vi "Solution part 1.vi"(11 "data?":bool) -> (3 "Distance":i32)   [LabVIEW 2020]
uses:
  Direction.ctl
  WindStar.ctl
panel:
  out "Non-90deg turn!":bool
  out "Last parsed line":i32
  out "Direction":T1
  out "Position":T2
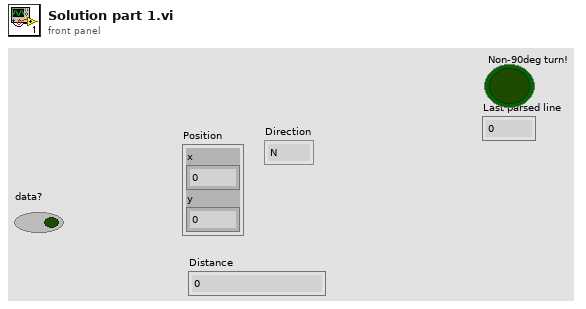
[diagram p1: front panel]
types:
  T1 = typedef "WindStar.ctl" = enum16{"N", "NE", "E", "SE", "S", "SW", "W", "NW", "F", "R", "L"}
  T2 = typedef "Direction.ctl" = cluster{"x":i32, "y":i32}
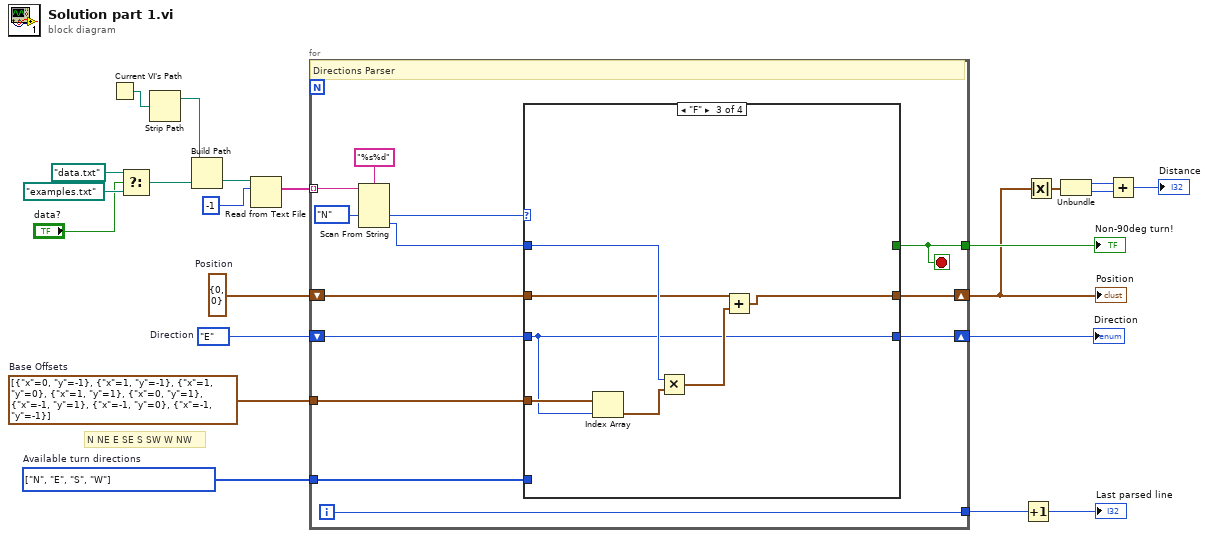
[diagram p0: block diagram]
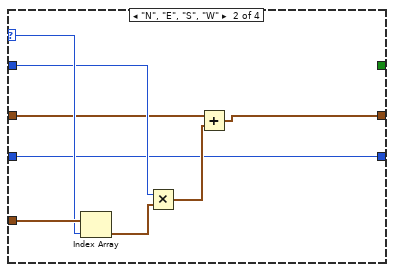
[diagram p3: hidden frame]
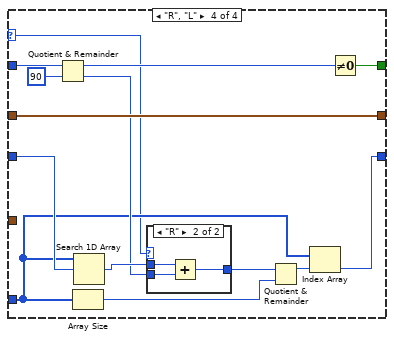
[diagram p4: hidden frame]
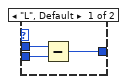
[diagram p5: hidden frame]
diagram:
  w9 = T1[] [enum."N", enum."E", enum."S", enum."W"] items=["N", "NE", "E", "SE", "S", "SW", "W", "NW", "F", "R", "L"]  # Available turn directions
  w13 = WindStar."E"  # Direction
  w11 = T2[] [{"x"=0, "y"=-1}, {"x"=1, "y"=-1}, {"x"=1, "y"=0}, {"x"=1, "y"=1}, {"x"=0, "y"=1}, {"x"=-1, "y"=1}, {"x"=-1, "y"=0}, {"x"=-1, "y"=-1}]  # Base Offsets
  w12 = T2 {"x"=0, "y"=0}  # Position
  # "N NE E SE S SW W NW"
  n1 = Current VI's Path() -> (path=w19:path)
  n2 = Select(t=path "data.txt", s="data?", f=path "examples.txt") -> (s? t:f=w20:path)
  n3 = Strip Path(path=w19) -> (stripped path=w18:path)  [unwired: 1 out]
  n4 = Build Path(base path=w18, name or relative path=w20) -> (appended path=w17:path)
  n5 = Read from Text File(file (use dialog)=w17, count=-1) -> (text=w14:string[])  [unwired: 2 in, 3 out]
  n6 = for {
    tunnel: w14 -> [w35] mode=indexing
    shift-right: [w28] -> w10
    shift-left: w13 -> [w32]
    shift-right: [w29] -> w5
    shift-left: w12 -> [w33]
    tunnel: w11 -> [w31]
    tunnel: w9 -> [w25]
    tunnel: [w24] -> w7
    tunnel: [w23] -> w8
    i -> [w23]
    stop <- w24 stop-if-true
    # "Directions Parser"
    n7 = Scan From String(format string="%s%d", input string=w35, default 1=WindStar."N") -> (output 1=w26:T1, output 2=w30:i32)  [unwired: 3 in, 3 out]
    n8 = case shown="\"F\"" w26 {
      selector: w26 -> [_ w44 _ w53]
      tunnel: w33 -> [w36 w41 w49 w66]
      tunnel: w32 -> [w37 w38 w46 w61]
      tunnel: w31 -> [_ w45 w52 _]
      tunnel: w30 -> [_ w42 w50 w65]
      tunnel: [w36 w39 w47 w66] -> w29
      tunnel: [w37 w38 w46 w54] -> w28
      tunnel: w25 -> [_ _ _ w55]
      tunnel: [_ _ _ w62] -> w24
      frame Default {
      }
      frame "N", "E", "S", "W" {
        n9 = Index Array(array=w45, index=w44) -> (element=w43:T2)
        n10 = Multiply(x=w42, y=w43) -> (x*y=w40:T2)
        n11 = Add(x=w41, y=w40) -> (x+y=w39:T2)
      }
      frame "F" {
        n12 = Index Array(array=w52, index=w46) -> (element=w51:T2)
        n13 = Multiply(x=w50, y=w51) -> (x*y=w48:T2)
        n14 = Add(x=w49, y=w48) -> (x+y=w47:T2)
      }
      frame "R", "L" {
        n15 = Quotient & Remainder(x=w65, y=90) -> (x-y*floor(x/y)=w63:i32, floor(x/y)=w59:i32)
        n16 = Array Size(array=w55) -> (size(s)=w57:i32)
        n17 = Search 1D Array(1D array=w55, element=w61) -> (index of element=w60:i32)  [unwired: 1 in]
        n18 = case shown="\"R\"" w53 {
          tunnel: w60 -> [w68 w72]
          tunnel: w59 -> [w69 w71]
          tunnel: [w67 w70] -> w58
          frame "L", Default {
            n19 = Subtract(x=w68, y=w69) -> (x-y=w67:i32)
          }
          frame "R" {
            n20 = Add(x=w72, y=w71) -> (x+y=w70:i32)
          }
        }
        n21 = Quotient & Remainder(x=w58, y=w57) -> (x-y*floor(x/y)=w56:i32)  [unwired: 1 out]
        n22 = Index Array(array=w55, index=w56) -> (element=w54:T1)
        n23 = Not Equal To 0?(x=w63) -> (x != 0?=w62:bool)
      }
    }
  }
  "Position" <- w5
  "Direction" <- w10
  "Non-90deg turn!" <- w7
  n24 = Increment(x=w8) -> (x+1=→"Last parsed line":i32)
  n25 = Absolute Value(x=w5) -> (abs(x)=w4:T2)
  n26 = Unbundle(w4) -> ("x"=w3:i32, "y"=w2:i32)
  n27 = Add(x=w3, y=w2) -> (x+y=→"Distance":i32)
